vi "InsertFirstNode.vi"(10 "New KD-Tree in":T1, 11 "Tree":dbl[](array[numeric])) -> (3 "New KD-Tree out":T1)   [LabVIEW 2016]
uses:
  KD-Tree.ctl
  Node.ctl
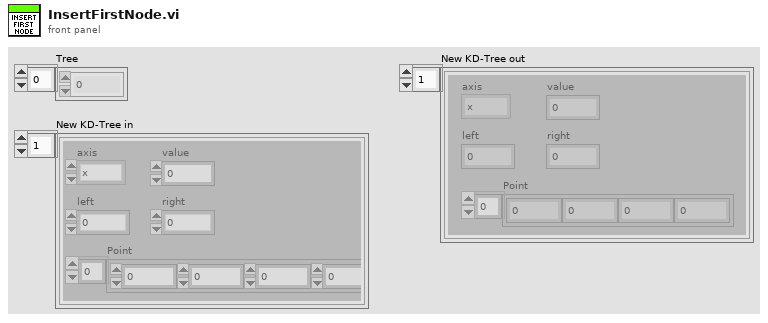
[diagram p1: front panel]
types:
  T1 = typedef "KD-Tree.ctl" = T2[]
  T2 = typedef "Node.ctl" = cluster{"axis":enum16{"null", "x", "y"}, "value":dbl, "left":dbl, "right":dbl, "Point":dbl[]}
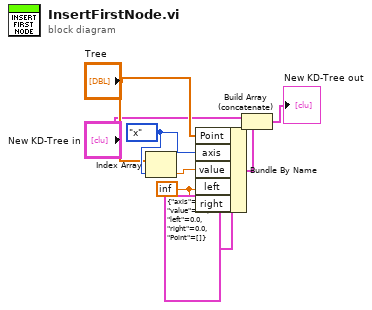
[diagram p0: block diagram]
diagram:
  w5 = inf
  w7 = enum16{"null", "x", "y"}."x" ("axis")
  n1 = Index Array(array="Tree", index=w7) -> (element=w8:dbl)
  n2 = Bundle By Name(cluster=T2 {"axis"=enum."x", "value"=0.0, "left"=0.0, "right"=0.0, "Point"=[]} ("element"), "Point"="Tree", "axis"=w7, "value"=w8, "left"=w5, "right"=w5) -> (w4:T2)
  n3 = Build Array (concatenate)("New KD-Tree in", w4) -> (→"New KD-Tree out":T1)
